vi "Memory.Pointer.Copy.Safe.vi"(8 "error in (no error)":errorcluster, 9 "bytes to copy":u64 format="%08x bytes", 10 "dst pointer in":refnum<class "Memory.Pointer.lvclass">, 11 "src pointer in":refnum<class "Memory.Pointer.lvclass">) -> (0 "error out":errorcluster, 1 "bytes to copy":u64 format="%08x bytes", 2 "dst pointer out":refnum<class "Memory.Pointer.lvclass">, 3 "src pointer out":refnum<class "Memory.Pointer.lvclass">)   [LabVIEW 2016, in "Memory Manager.lvlib" / "Memory.Pointer.lvclass"]
doc: "Copies a specified subset of the data stored at the memory location of the <b>src pointer</b> into the memory address associated with <b>dst pointer</b>.\n\n<b>Note:</b> This VI is <b>safe</b>.\n\nSafe means that this function evaluates that the size parameter of <b>dst pointer</b> is greater than or equal to the size of the requested memory from <b>src pointer</b> to ensure that the destination memory location is an appropriate size before copying data from source to destination. Reading/writing more data to a pointer than it has allocated can corrupt or crash LabVIEW."
uses:
  Memory.Pointer.lvclass
  Memory.Pointer.lvclass/Memory.Pointer.ctl
  Accessors/Get Address.vi
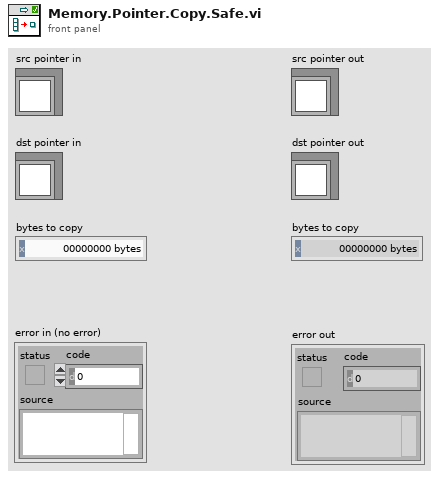
[diagram p1: front panel]
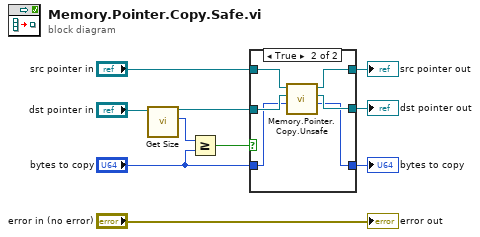
[diagram p0: block diagram]
diagram:
  n1 = call "Get Size.vi"("Pointer in"="dst pointer in") -> ("size"=w9:u64, "Pointer out"=w5:refnum<class "Memory.Pointer.lvclass">)  [unwired: 8 in, 1 out]
  n2 = Greater Or Equal?(x=w9, y="bytes to copy") -> (x >= y?=w8:bool)
  n3 = case shown="True" w8 {
    tunnel: [w11 w14] -> w7
    tunnel: "bytes to copy" -> [w11 w15]
    tunnel: "src pointer in" -> [w13 w19]
    tunnel: w5 -> [w12 w18]
    tunnel: [w13 w17] -> w4
    tunnel: [w12 w16] -> w3
    frame False {
    }
    frame True {
      n4 = call "Memory.Pointer.Copy.Unsafe.vi"("bytes to copy"=w15, "dst pointer in"=w18, "src pointer in"=w19) -> ("bytes to copy"=w14:u64, "dst pointer out"=w16:refnum<class "Memory.Pointer.lvclass">, "src pointer out"=w17:refnum<class "Memory.Pointer.lvclass">)  [unwired: 5 in, 1 out]
    }
  }
  "src pointer out" <- w4
  "dst pointer out" <- w3
  "bytes to copy" <- w7
  "error out" <- "error in (no error)"
